vi "Main.vi"() -> ()   [LabVIEW 2026]
doc: "============================================================\nPI-C867-IO Control — VI Principal\nVersion : 0.0\nDate : Avril 2026\nAuteur : Institut Fresnel / Photonics Platform\n============================================================\n\nDESCRIPTION\n-----------\nVI de pilotage multi-positions du contrôleur PI C-867 pour\nmicroscopie de polarisation. Gère la séquence de déplacement\nXY synchronisée avec l'acquisition (lasers, polariseurs, caméra)\nvia signaux TTL hardware sans dialogue RS-232 pendant la DAQ.\n\nFACE AVANT\n----------\nEntrées :\n - Tableau XY (Nx2 DBL) : positions en mm\n - Nb boucles (I32) : nombre de répétitions de la séquence\n - Bouton Go : démarre la séquence\n - Bouton Stop : arrêt immédiat\n\nIndicateurs :\n - Position courante : ex. \"3 / 5\"\n - Boucle courante : ex. \"2 / 3\"\n - État : message texte (Initialisé / En cours / Arrêté)\n - Erreur : code et description\n\nMACHINE À ÉTATS\n---------------\nINIT ? Connexion C-867 (USB), SVO, FRF\n Init task CO (GO) et task DI (READY)\nWAIT_FOR_EVENT ? Attente bouton Go ou Quitter\nLOAD_POSITIONS ? Envoi macro via Python (main.py)\nRUNNING ? Émission impulsion GO (compteur CO)\nWAIT_READY ? Attente front montant READY (Change Detection)\nACQUIRE ? Acquisition (1s en test) + gestion boucles\nSTOP ? Arrêt C-867, clear tasks DAQ\n\nCONNEXIONS HARDWARE\n-------------------\nC-867 broche 4 (jaune) ? PFI13 Dev USB-6353-3 (GO)\nC-867 broche 5 (violet) ? P0.4 Dev USB-6353-3 (READY)\nGND (blindage) ? DGND\n\nDÉPENDANCES\n-----------\n- PI GCS LabVIEW VIs (C:\\ProgramData\\PI\\LabVIEW\\)\n- Python 3.x + PIPython\n- Scripts : main.py, macro_builder.py\n- NI-DAQmx\n============================================================"
uses:
  SubVI/Controls/Etats.ctl
  SubVI/Controls/TypeDef_FGV.ctl
  <vilib>/DAQmx/read.llb/DAQmx Read (Digital Bool 1Line 1Point).vi
  <vilib>/DAQmx/miscellaneous.llb/DAQmx Fill In Error Info.vi
panel:
  out "Current loop":u32=1
  out "Current pos":i32=1
  in  "Emergency stop":bool
  in  "# of Loops":dbl=3.0
  in  "Position table":dbl[][](array[numeric])=[[0.0, 0.0, 0.0], [0.1, 0.1, 0.0], [0.2, 0.2, 0.0], [0.3, 0.3, 0.0], [0.1, 0.2, 0.0]]
  out "error out":errorcluster caption="sortie d'erreur"
  in  "error in":errorcluster caption="entrée d'erreur"
  in  "Arrêter":bool
  in  "GO":bool
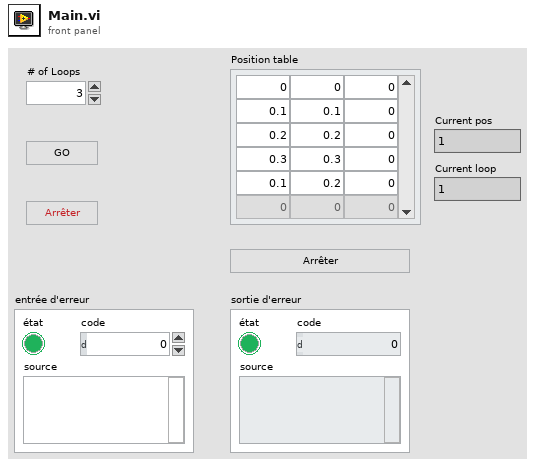
[diagram p1: front panel]
types:
  T1 = typedef "TypeDef_FGV.ctl" = enum16{"Initialize", "Write", "Read"}
  T2 = typedef "Etats.ctl" = enum16{"INIT", "WAIT_FOR_EVENT", "LOAD_POSITIONS", "RUNNING", "WAIT_READY", "ACQUIRE", "STOP"}
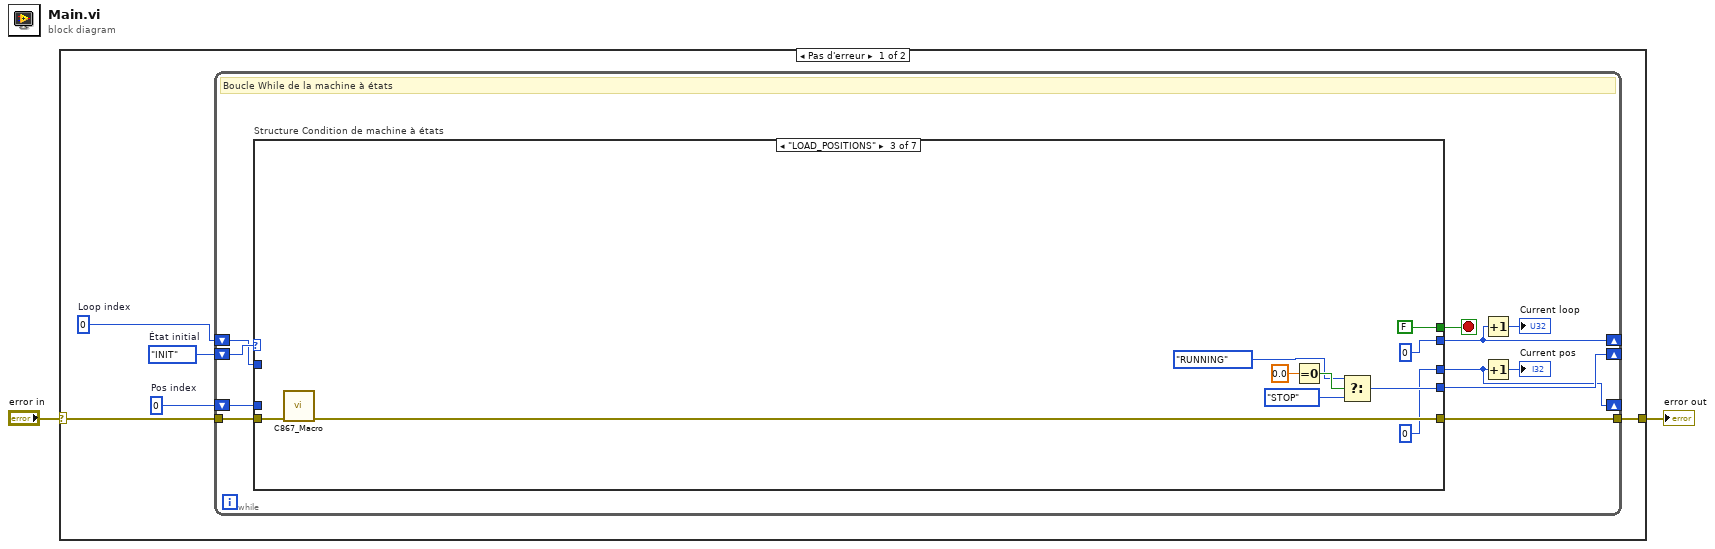
[diagram p0: block diagram]
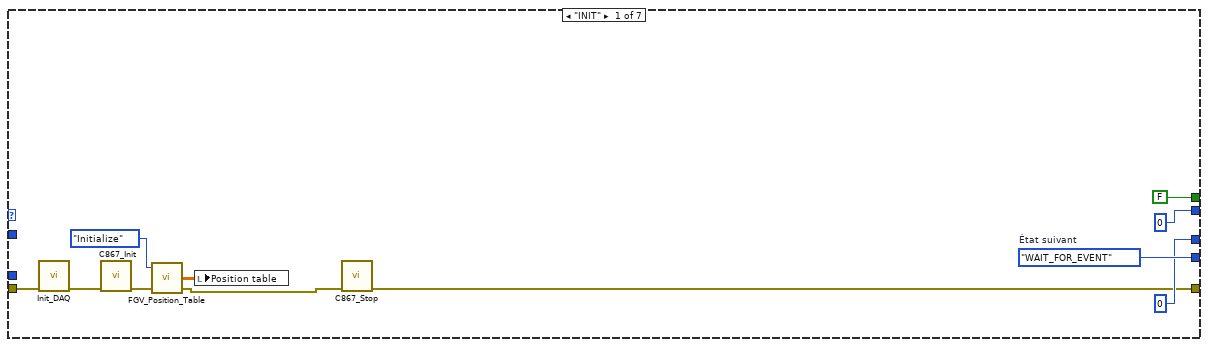
[diagram p2: hidden frame]
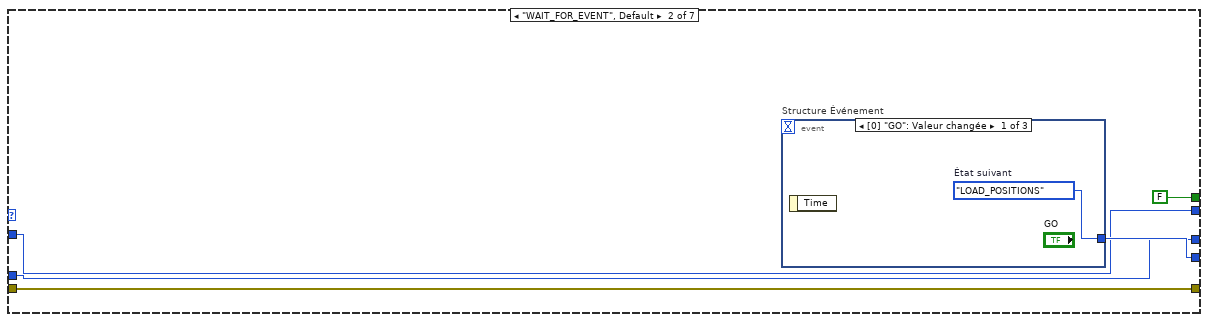
[diagram p3: hidden frame]
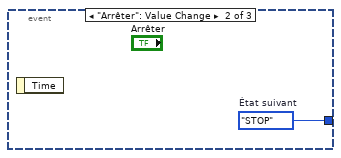
[diagram p4: hidden frame]
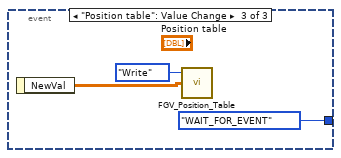
[diagram p5: hidden frame]
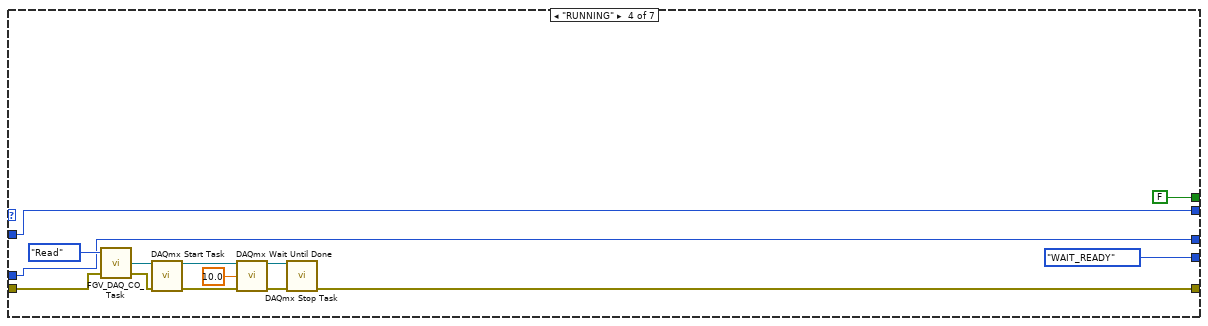
[diagram p6: hidden frame]
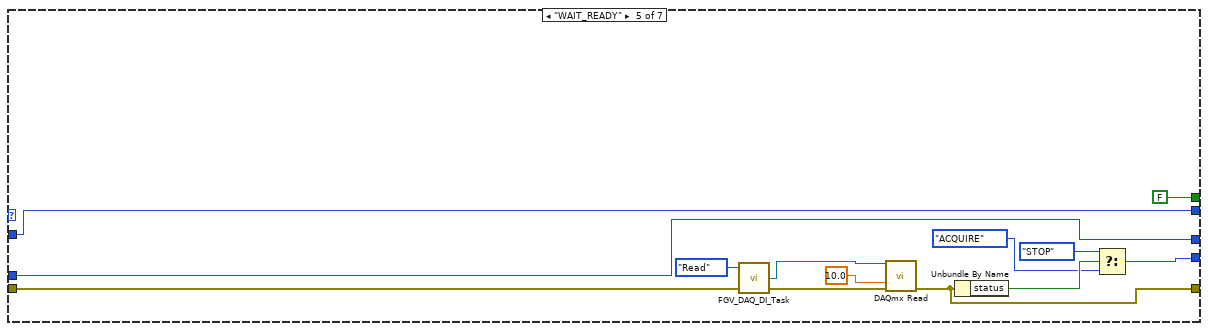
[diagram p7: hidden frame]
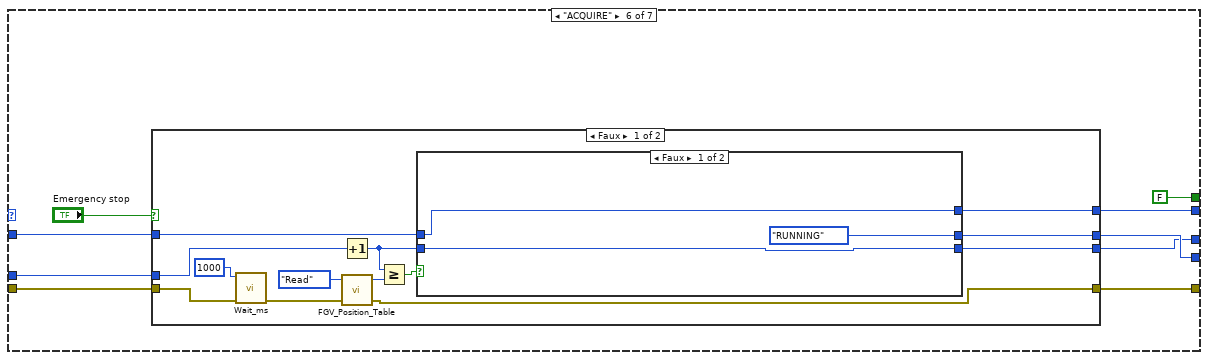
[diagram p8: hidden frame]
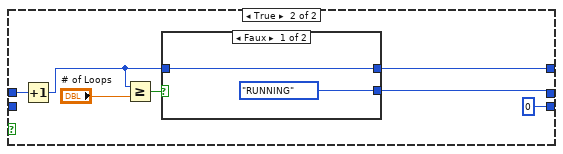
[diagram p9: hidden frame]
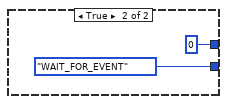
[diagram p10: hidden frame]
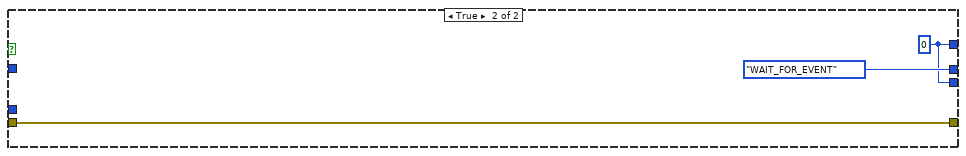
[diagram p11: hidden frame]
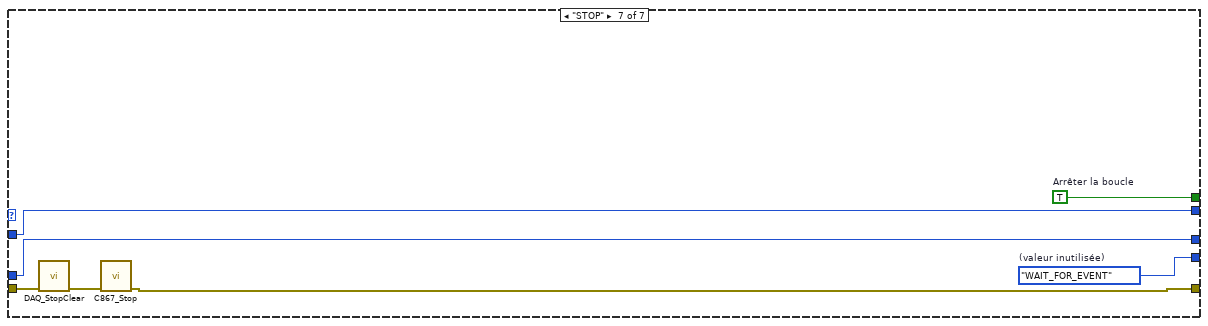
[diagram p12: hidden frame]
diagram:
  n1 = case shown="Pas d'erreur" "error in" {
    selector: "error in" -> [w6 w123]
    tunnel: [w5 w123] -> w1
    frame No Error {
      w3 = 0  # Loop index
      w4 = 0  # Pos index
      w7 = Etats."INIT"  # État initial
      n2 = while {
        shift-right: [w17] -> _
        shift-left: w7 -> [w18]
        tunnel: w6 -> [w15]
        tunnel: [w14] -> w5
        shift-right: [w13] -> _
        shift-left: w4 -> [w11]
        shift-right: [w12] -> _
        shift-left: w3 -> [w10]
        stop <- w16 stop-if-true
        # "Boucle While de la machine à états"
        n3 = case "Structure Condition de machine à états" shown="\"LOAD_POSITIONS\"" w18 {
          tunnel: [w29 w34 w43 Etats."WAIT_READY" ("(valeur inutilisée)") w68 w81 w122] -> w17
          tunnel: [FALSE ("Arrêter la boucle") FALSE ("Arrêter la boucle") FALSE ("Arrêter la boucle") FALSE ("Arrêter la boucle") FALSE ("Arrêter la boucle") FALSE ("Arrêter la boucle") w121] -> w16
          tunnel: w15 -> [w27 w32 w48 w58 w75 w83 w120]
          tunnel: [w19 w32 w47 w52 w71 w82 w116] -> w14
          tunnel: [0 ("Pos index") w31 0 ("Pos index") w51 w65 w80 w119] -> w13
          tunnel: [u32 0 ("milliseconds to wait") w30 u32 0 ("milliseconds to wait") w50 w64 w79 w118] -> w12
          tunnel: w11 -> [_ w31 _ w51 w65 w78 w119]
          tunnel: w10 -> [_ w30 _ w50 w64 w77 w118]
          frame "INIT" {
            w29 = Etats."WAIT_FOR_EVENT"  # État suivant
            n4 = call "Init_DAQ.vi"("error in"=w27) -> ("error out"=w26:errorcluster)  [unwired: 10 in]
            n5 = call "C867_Init.vi"("error in"=w26) -> ("error out"=w23:errorcluster)  [unwired: 9 in, 1 out]
            n6 = call "FGV_Position_Table.vi"("error in"=w23, "Action"=TypeDef_FGV."Initialize") -> ("error out"=w20:errorcluster, "Position table"=w21:dbl[][])  [unwired: 1 in, 1 out]
            n7 = local write "Position table"(w21) -> ()
            n8 = call "C867_Stop.vi"("error in"=w20) -> ("error out"=w19:errorcluster)  [unwired: 10 in]
          }
          frame "WAIT_FOR_EVENT", Default {
            n9 = event "Structure Événement" shown="[0] \"GO\": Valeur changée" {
              selector: _ -> [_ _ _]
              dyn-events: _ -> [_ _ _]
              timeout: _ -> [_ _ _]
              tunnel: [w35 w36 Etats."WAIT_FOR_EVENT" ("État suivant")] -> w34
              event "GO": Value Change {
                w35 = Etats."LOAD_POSITIONS"  # État suivant
                n10 = event-data() -> ()  [unwired: 1 in, 1 out]
              }
              event "Arrêter": Value Change {
                w36 = Etats."STOP"  # État suivant
                n11 = event-data() -> ()  [unwired: 1 in, 1 out]
              }
              event "Position table": Value Change {
                n12 = event-data() -> ("NewVal"=w39:dbl[][])  [unwired: 1 in]
                n13 = call "FGV_Position_Table.vi"("Position table"=w39, "Action"=TypeDef_FGV."Write") -> ()  [unwired: 1 in, 3 out]
              }
            }
          }
          frame "LOAD_POSITIONS" {
            n14 = call "C867_Macro.vi"("error in"=w48) -> ("error out"=w47:errorcluster)  [unwired: 10 in]
            n15 = Equal To 0?(x=0.0) -> (x = 0?=w46:bool)
            n16 = Select(t=Etats."RUNNING" ("(valeur inutilisée)"), s=w46, f=Etats."STOP" ("cas faux")) -> (s? t:f=w43:T2)
          }
          frame "RUNNING" {
            n17 = call "FGV_DAQ_CO_Task.vi"("error in"=w58, "Action"=TypeDef_FGV."Read") -> ("error out"=w61:errorcluster, "CO task"=w60:refnum<k21>)  [unwired: 2 in]
            n18 = call <vilib>:"DAQmx Start Task.vi"("task/channels in"=w60, "error in"=w61) -> ("task out"=w57:refnum<k21>, "error out"=w55:errorcluster)  [unwired: 12 in]
            n19 = call <vilib>:"DAQmx Wait Until Done.vi"("task/channels in"=w57, "timeout (sec)"=10.0, "error in"=w55) -> ("task out"=w54:refnum<k21>, "error out"=w53:errorcluster)  [unwired: 11 in]
            n20 = call <vilib>:"DAQmx Stop Task.vi"("task/channels in"=w54, "error in"=w53) -> ("error out"=w52:errorcluster)  [unwired: 12 in, 1 out]
          }
          frame "WAIT_READY" {
            n21 = call "FGV_DAQ_DI_Task.vi"("error in"=w75, "Action"=TypeDef_FGV."Read") -> ("error out"=w74:errorcluster, "DI task"=w73:refnum<k21>)  [unwired: 2 in]
            n22 = call-poly <vilib>:"DAQmx Read.vi"("task/channels in"=w73, "timeout"=10.0, "error in"=w74) -> ("error out"=w71:errorcluster)  [unwired: 10 in, 2 out]
            n23 = Unbundle By Name(w71) -> ("status"=w70:bool)
            n24 = Select(t=Etats."STOP" ("(valeur inutilisée)"), s=w70, f=Etats."ACQUIRE" ("(valeur inutilisée)")) -> (s? t:f=w68:T2)
          }
          frame "ACQUIRE" {
            n25 = case shown="Faux" "Emergency stop" {
              tunnel: w83 -> [w97 w114]
              tunnel: [w93 w114] -> w82
              tunnel: [w91 Etats."WAIT_FOR_EVENT" ("(valeur inutilisée)")] -> w81
              tunnel: [w89 w113] -> w80
              tunnel: [w88 w113] -> w79
              tunnel: w78 -> [w90 _]
              tunnel: w77 -> [w87 _]
              frame False {
                n26 = call "Wait_ms.vi"("error in (no error)"=w97, "milliseconds to wait"=u32 1000) -> ("error out"=w95:errorcluster)  [unwired: 9 in]
                n27 = Increment(x=w90) -> (x+1=w92:i32)
                n28 = call "FGV_Position_Table.vi"("error in"=w95, "Action"=TypeDef_FGV."Read") -> ("error out"=w93:errorcluster, "N pos"=w86:i32)  [unwired: 1 in, 1 out]
                n29 = Greater Or Equal?(x=w92, y=w86) -> (x >= y?=w96:bool)
                n30 = case shown="Faux" w96 {
                  tunnel: w92 -> [w100 _]
                  tunnel: [Etats."RUNNING" ("(valeur inutilisée)") w106] -> w91
                  tunnel: [w100 0] -> w89
                  tunnel: [w99 w103] -> w88
                  tunnel: w87 -> [w99 w102]
                  frame False {
                  }
                  frame True {
                    n31 = Increment(x=w102) -> (x+1=w105:u32)
                    n32 = Greater Or Equal?(x=w105, y="# of Loops") -> (x >= y?=w107:bool)
                    n33 = case shown="Faux" w107 {
                      tunnel: [w109 u32 0 ("milliseconds to wait")] -> w103
                      tunnel: [Etats."RUNNING" ("(valeur inutilisée)") Etats."WAIT_FOR_EVENT" ("(valeur inutilisée)")] -> w106
                      tunnel: w105 -> [w109 _]
                      frame False {
                      }
                      frame True {
                      }
                    }
                  }
                }
              }
              frame True {
                w113 = 0
              }
            }
          }
          frame "STOP" {
            w121 = TRUE  # Arrêter la boucle
            w122 = Etats."WAIT_FOR_EVENT"  # (valeur inutilisée)
            n34 = call "DAQ_StopClear.vi"("error in"=w120) -> ("error out"=w117:errorcluster)  [unwired: 10 in]
            n35 = call "C867_Stop.vi"("error in"=w117) -> ("error out"=w116:errorcluster)  [unwired: 10 in]
          }
        }
        n36 = Increment(x=w12) -> (x+1=→"Current loop":u32)
        n37 = Increment(x=w13) -> (x+1=→"Current pos":i32)
      }
    }
    frame Error {
    }
  }
  "error out" <- w1
